vi "Begin.vi"(8 "error in (no error)":errorcluster, 11 "Xbox Controller-Physical in":refnum<class "Xbox Controller-Physical.lvclass">) -> (0 "error out":errorcluster, 3 "Xbox Controller-Physical out":refnum<class "Xbox Controller-Physical.lvclass">)   [LabVIEW 2013, in "Physical Systems.lvlib" / "XBox Controller.lvlib" / "Xbox Controller-Physical.lvclass"]
uses:
  Xbox Controller-Physical.lvclass
  <vilib>/Rock Robotics/WPI/Joystick/WPI_JoystickDeviceEnum.ctl
  Xbox Controller-Physical.lvclass/Xbox Controller-Physical.ctl
  Virtual Systems/XBox Controller/XBox Controller Class/XBox Controller-Logical.lvclass
panel:
  in  "JoystickDevice":T1
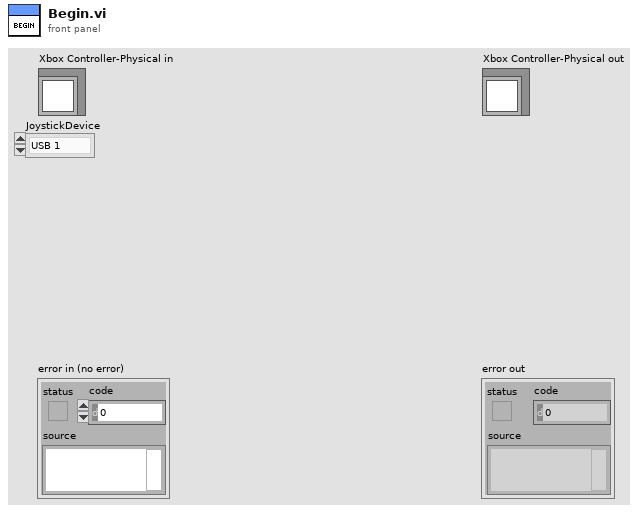
[diagram p1: front panel]
types:
  T1 = typedef "WPI_JoystickDeviceEnum.ctl" = enum16{"USB 1", "USB 2", "USB 3", "USB 4", "Kinect 1", "Kinect 2"}
  T2 = typedef "WPI_JoystickDevRef.ctl" = cluster{"Device":T1}
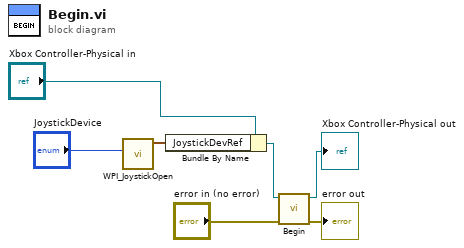
[diagram p0: block diagram]
diagram:
  n1 = call <vilib>:"WPI_JoystickOpen.vi"("JoystickDevice"="JoystickDevice") -> ("JoystickDevRef"=w1:T2)  [unwired: 10 in]
  n2 = Bundle By Name(cluster="Xbox Controller-Physical in", "JoystickDevRef"=w1) -> (w2:refnum<class "Xbox Controller-Physical.lvclass">)
  n3 = call-parent "Begin.vi"("error in (no error)"="error in (no error)", "System Actor in"=w2) -> ("error out"=→"error out":errorcluster, "System Actor out"=→"Xbox Controller-Physical out":refnum<class "Xbox Controller-Physical.lvclass">)  [unwired: 8 in]
